vi "Stages.GetValues.vi"(8 "error in (no error)":errorcluster, 11 "Async Parameters in":T1) -> (0 "error out":errorcluster, 3 "Async Parameters out":T1)   [LabVIEW 2019, in "Fuel Injector Analysis Addon Engine.lvlib"]
uses:
  Fuel Injector Analysis Addon Engine.lvlib
  Types/Async Parameters.ctl
  Addon Shared/Types/Shot.Parameters.ctl
  Addon Shared/Types/Stage.Parameters.ctl
  Addon Shared/Types/Stage.PullIn.Types.ctl
  Addon Shared/Types/Stage.Transition.Types.ctl
  Addon Shared/Types/Analysis.Channels.Select.ctl
  Addon Shared/Types/Injector info.ctl
  Types/Injector.State.ctl
  <vilib>/NI/NIVS Inline Async API/_Data Access Engine/Data Access Engine/Types/Write.DVR.ctl
  <vilib>/NI/NIVS Inline Async API/_Data Access Engine/Access Type Classes/Write/Write.lvclass
  <vilib>/NI/NIVS Inline Async API/_Data Access Engine/Data Access Engine/Types/Read.DVR.ctl
  <vilib>/NI/NIVS Inline Async API/_Data Access Engine/Access Type Classes/Read/Read.lvclass
  Addon Shared/Types/Compiled.Group.WaveformRefs.ctl
  <vilib>/NI VeriStand/Custom Device API/Waveform Data Reference.ctl
  <vilib>/NI VeriStand/Custom Device Waveform API/Single Waveform Write (DBL)/Single Waveform Write (DBL).lvclass
  <vilib>/NI/NIVS Inline Async API/_Data Access Engine/Access Type Classes/Read/Read.lvclass/Read.ctl
  <vilib>/NI/NIVS Inline Async API/_Data Access Engine/Data Access Engine/Methods/Read.Data.vi
  <vilib>/NI/NIVS Inline Async API/_Data Access Engine/Access Type Classes/Read/Read.ProcessData.vi
  Addon Shared/SubVIs/Constants.vi
  <vilib>/NI/NIVS Inline Async API/_Data Access Engine/Data Access Engine/Data Access Engine.lvclass
  Addon Shared/Fuel Injector Analysis Addon Shared.lvlib
  <vilib>/NI VeriStand/Custom Device API/Custom Device API.lvlib
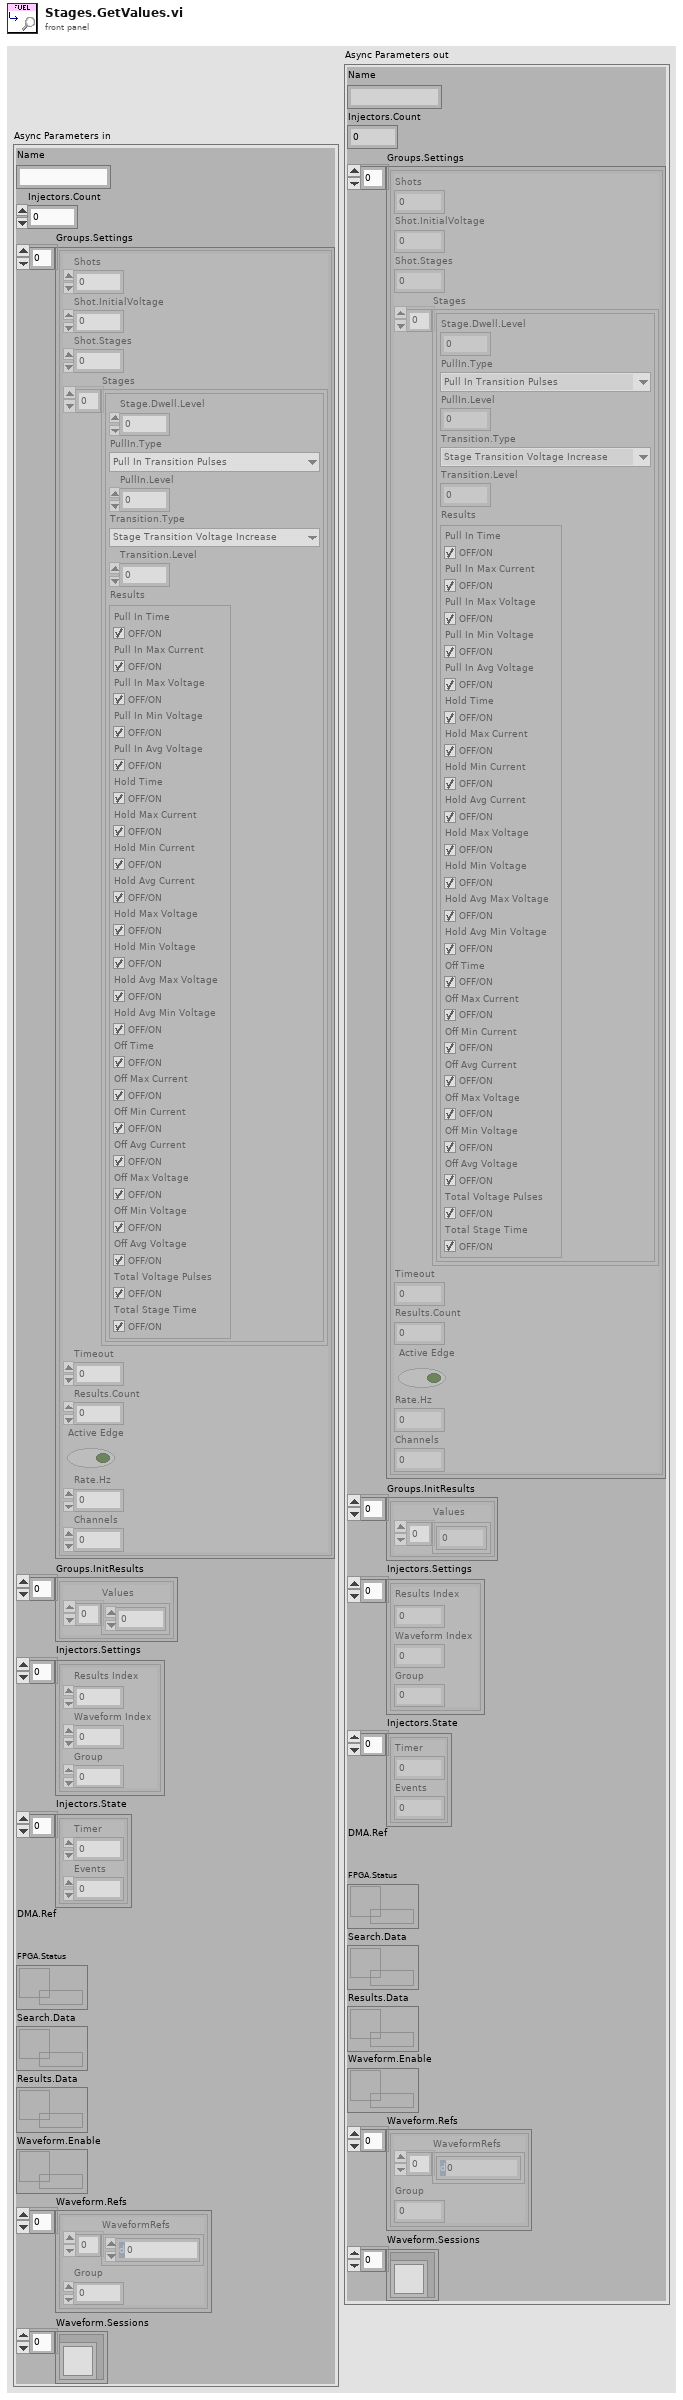
[diagram p1: front panel]
types:
  T1 = typedef "Fuel Injector Analysis Addon Engine.lvlib/Async Parameters.ctl" = cluster{"Name":string, "Injectors.Count":u8, "Groups.Settings":T2[], "Groups.InitResults":cluster{"Values":dbl[]}[], "Injectors.Settings":T7[], "Injectors.State":T8[], "DMA.Ref":refnum<k20>, "FPGA.Status":T9, "Search.Data":T10, "Results.Data":T9, "Waveform.Enable":T10, "Waveform.Refs":T11[], "Waveform.Sessions":refnum<class "Single Waveform Write (DBL).lvclass">[]}
  T2 = typedef "Fuel Injector Analysis Addon Shared.lvlib/Shot.Parameters.ctl" = cluster{"Shots":u32, "Shot.InitialVoltage":dbl, "Shot.Stages":u32, "Stages":T3[], "Timeout":dbl, "Results.Count":i32, "Active Edge":bool, "Rate.Hz":u32, "Channels":u32}
  T3 = typedef "Fuel Injector Analysis Addon Shared.lvlib/Stage.Parameters.ctl" = cluster{"Stage.Dwell.Level":dbl, "PullIn.Type":T4, "PullIn.Level":dbl, "Transition.Type":T5, "Transition.Level":dbl, "Results":T6}
  T4 = typedef "Fuel Injector Analysis Addon Shared.lvlib/Stage.PullIn.Types.ctl" = enum8{"Pull In Transition Pulses", "Pull In Transition Current Drop"}
  T5 = typedef "Fuel Injector Analysis Addon Shared.lvlib/Stage.Transition.Types.ctl" = enum8{"Stage Transition Inactive Time", "Stage Transition Voltage Increase", "Stage Transition Current Decrease", "Stage Transition Active Time"}
  T6 = typedef "Fuel Injector Analysis Addon Shared.lvlib/Analysis.Channels.Select.ctl" = cluster{"Pull In Time":bool, "Pull In Max Current":bool, "Pull In Max Voltage":bool, "Pull In Min Voltage":bool, "Pull In Avg Voltage":bool, "Hold Time":bool, "Hold Max Current":bool, "Hold Min Current":bool, "Hold Avg Current":bool, "Hold Max Voltage":bool, "Hold Min Voltage":bool, "Hold Avg Max Voltage":bool, "Hold Avg Min Voltage":bool, "Off Time":bool, "Off Max Current":bool, "Off Min Current":bool, "Off Avg Current":bool, "Off Max Voltage":bool, "Off Min Voltage":bool, "Off Avg Voltage":bool, "Total Voltage Pulses":bool, "Total Stage Time":bool}
  T7 = typedef "Fuel Injector Analysis Addon Shared.lvlib/Injector info.ctl" = cluster{"Results Index":i32, "Waveform Index":i32, "Group":u16}
  T8 = typedef "Fuel Injector Analysis Addon Engine.lvlib/Injector.State.ctl" = cluster{"Timer":u32, "Events":u64}
  T9 = typedef "Data Access Engine.lvlib/Data Access Engine.lvclass/Write.DVR.ctl" = refnum<data-value>
  T10 = typedef "Data Access Engine.lvlib/Data Access Engine.lvclass/Read.DVR.ctl" = refnum<data-value>
  T11 = typedef "Fuel Injector Analysis Addon Shared.lvlib/Compiled.Group.WaveformRefs.ctl" = cluster{"WaveformRefs":T12[], "Group":i32}
  T12 = typedef "Custom Device API.lvlib/Waveform Data Reference.ctl" = i32
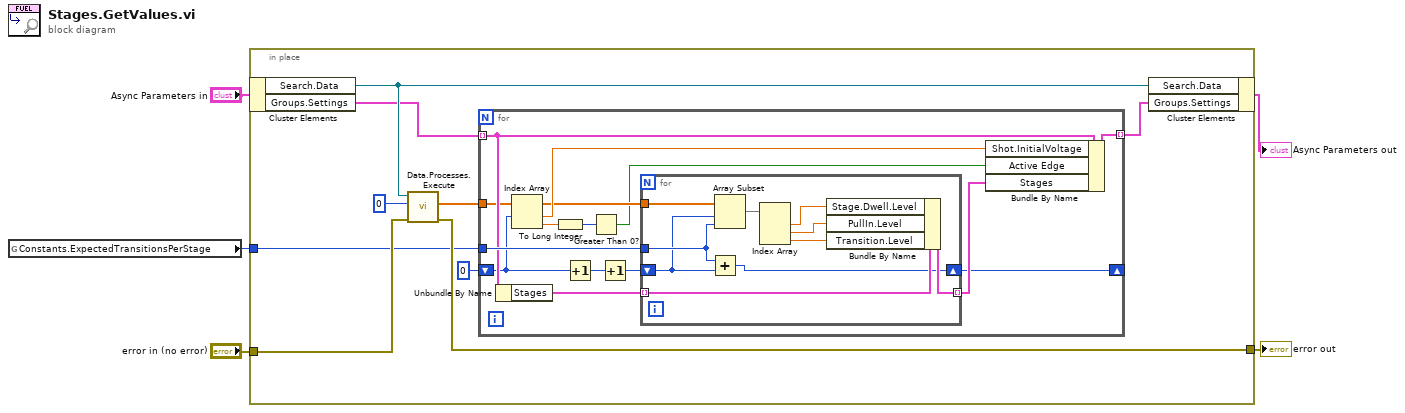
[diagram p0: block diagram]
diagram:
  n1 = global read "Constants.vi" "Constants.ExpectedTransitionsPerStage"() -> (w1:u32)
  n2 = in-place {
    in-place-border: "error in (no error)" -> [w13]
    in-place-border: [w12] -> w5
    in-place-border: w1 -> [w11]
    n3 = in-place-cluster #1("Async Parameters in") -> ("Search.Data"=w14:T10, "Groups.Settings"=w10:T2[])
    n4 = call-poly <vilib>:"Data.Processes.Execute.vi"("error in (no error)"=w13, "timeout ms"=0 ("timeout in ms (0)"), "Ref"=w14) -> ("error out"=w12:errorcluster, "Values"=w7:dbl[])  [unwired: 6 in, 1 out]
    n5 = for {
      tunnel: w11 -> [w28]
      tunnel: w10 -> [w24] mode=indexing
      tunnel: [w27] -> w9 mode=indexing
      tunnel: w7 -> [w22]
      shift-right: [w21] -> _
      shift-left: u32 0 -> [w20]
      n6 = Unbundle By Name(w24) -> ("Stages"=w23:T3[])
      n7 = Index Array(array=w22, index #1=w20) -> (element #1=w26:dbl, element #2=w17:dbl)  [unwired: 1 in]
      n8 = To Long Integer(number=w17) -> (32bit integer=w16:i32)
      n9 = Increment(x=w20) -> (x+1=w19:u32)
      n10 = Greater Than 0?(x=w16) -> (x > 0?=w15:bool)
      n11 = Increment(x=w19) -> (x+1=w18:u32)
      n12 = for {
        tunnel: w23 -> [w38] mode=indexing
        tunnel: [w37] -> w25 mode=indexing
        tunnel: w22 -> [w36]
        tunnel: w28 -> [w31]
        shift-right: [w29] -> w21
        shift-left: w18 -> [w30]
        n13 = Add(x=w31, y=w30) -> (x+y=w29:u32)
        n14 = Array Subset(array=w36, index=w30, length=w31) -> (w35:dbl[])
        n15 = Index Array(array=w35) -> (element #1=w34:dbl, element #2=w33:dbl, element #3=w32:dbl)  [unwired: 3 in]
        n16 = Bundle By Name(cluster=w38, "Stage.Dwell.Level"=w34, "PullIn.Level"=w33, "Transition.Level"=w32) -> (w37:T3)
      }
      n17 = Bundle By Name(cluster=w24, "Shot.InitialVoltage"=w26, "Active Edge"=w15, "Stages"=w25) -> (w27:T2)
    }
    n18 = in-place-cluster #1("Search.Data"=w14, "Groups.Settings"=w9) -> (→"Async Parameters out":T1)
  }
  "error out" <- w5
